vi "generate command value.vi"(8 "data":u8, 9 "index":u8, 10 "device":u8, 11 "action":T1) -> (3 "Element":u32)   [LabVIEW 2013, in "dynamic profibus.lvlib"]
uses:
  dynamic profibus.lvlib
  profibus master action.ctl
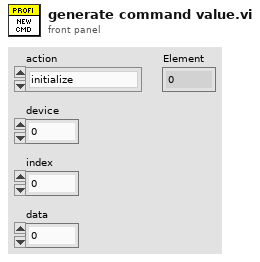
[diagram p1: front panel]
types:
  T1 = typedef "dynamic profibus.lvlib/profibus master action.ctl" = enum8{"initialize", "uninitialize", "stop", "get input", "get input size", "set output", "get output size", "get diagnostic", "transfer data", "transfer diagnostics", "read many inputs"}
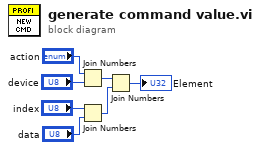
[diagram p0: block diagram]
diagram:
  n1 = Join Numbers(hi="action", lo="device") -> ((hi.lo)=w6:u16)
  n2 = Join Numbers(hi="index", lo="data") -> ((hi.lo)=w7:u16)
  n3 = Join Numbers(hi=w6, lo=w7) -> ((hi.lo)=→"Element":u32)
